vi "SO-PPSU TDK Lambda Voltage update.vi"(7 "queue In":refnum<queue>, 8 "error In":errorcluster, 9 "Ramp  time(sec)":dbl, 10 "connection ID":refnum<k5>, 11 "Voltage":string) -> (0 "error out":errorcluster, 1 "Boolean":bool, 2 "connection ID 3":refnum<k5>, 4 "PPSU OUT PUT":T1, 5 "queue In 2":refnum<queue>)   [LabVIEW 2022 SP3]
uses:
  <vilib>/ptbypt/NI_PtbyPt.lvlib
  <vilib>/Analysis/NI_AALBase.lvlib
  Controls/FGV Read write.ctl
  <vilib>/Analysis/1siggen.llb/Ramp Pattern by Samples.vi
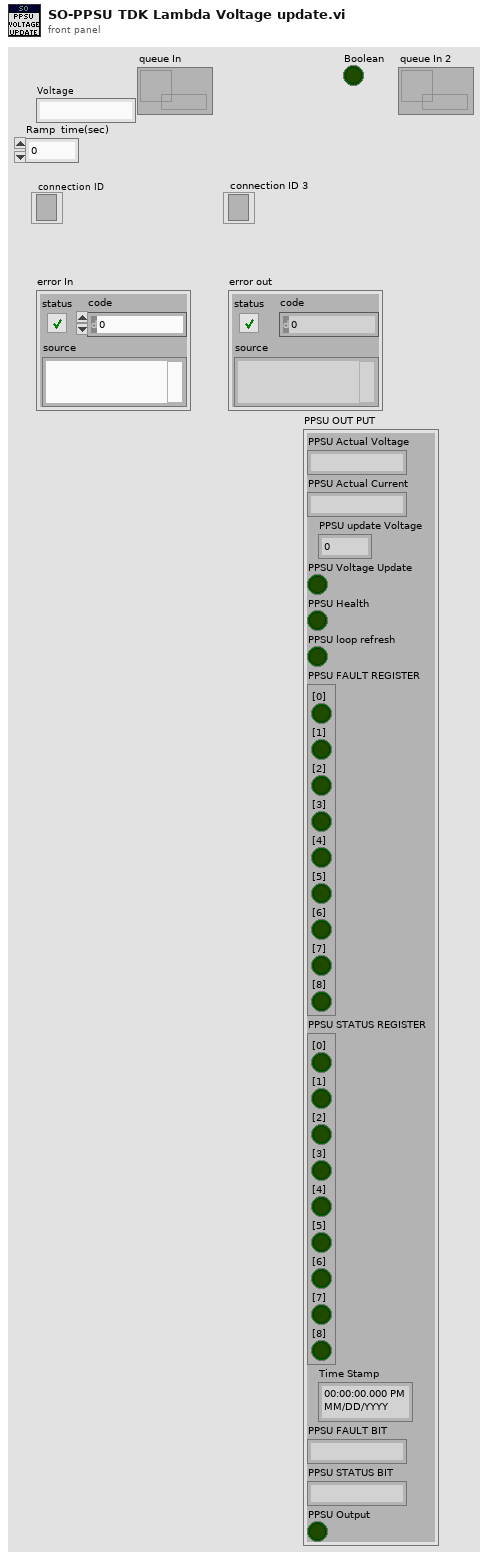
[diagram p1: front panel]
types:
  T1 = cluster{"PPSU Actual Voltage ":string, "PPSU Actual Current ":string, "PPSU update Voltage ":dbl, "PPSU Voltage Update":bool, "PPSU Health":bool, "PPSU loop refresh":bool, "PPSU FAULT REGISTER":cluster{"[0]":bool, "[1]":bool, "[2]":bool, "[3]":bool, "[4]":bool, "[5]":bool, "[6]":bool, "[7]":bool, "[8]":bool}, "PPSU STATUS REGISTER":cluster{"[0]":bool, "[1]":bool, "[2]":bool, "[3]":bool, "[4]":bool, "[5]":bool, "[6]":bool, "[7]":bool, "[8]":bool}, "Time Stamp":timestamp, "PPSU FAULT BIT":string, "PPSU STATUS BIT ":string, "PPSU Output":bool}
  T2 = typedef "FGV Read write.ctl" = enum16{"Write", "Read"}
  T3 = cluster{"[0]":bool, "[1]":bool, "[2]":bool, "[3]":bool, "[4]":bool, "[5]":bool, "[6]":bool, "[7]":bool, "[8]":bool}
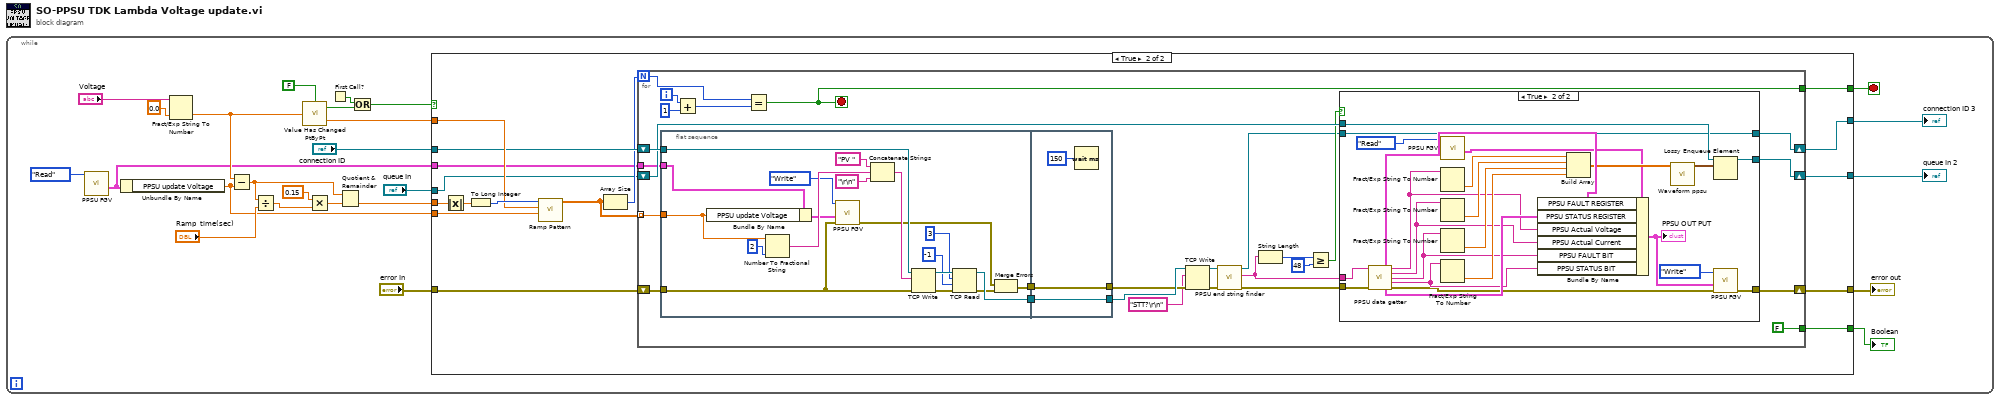
[diagram p0: block diagram]
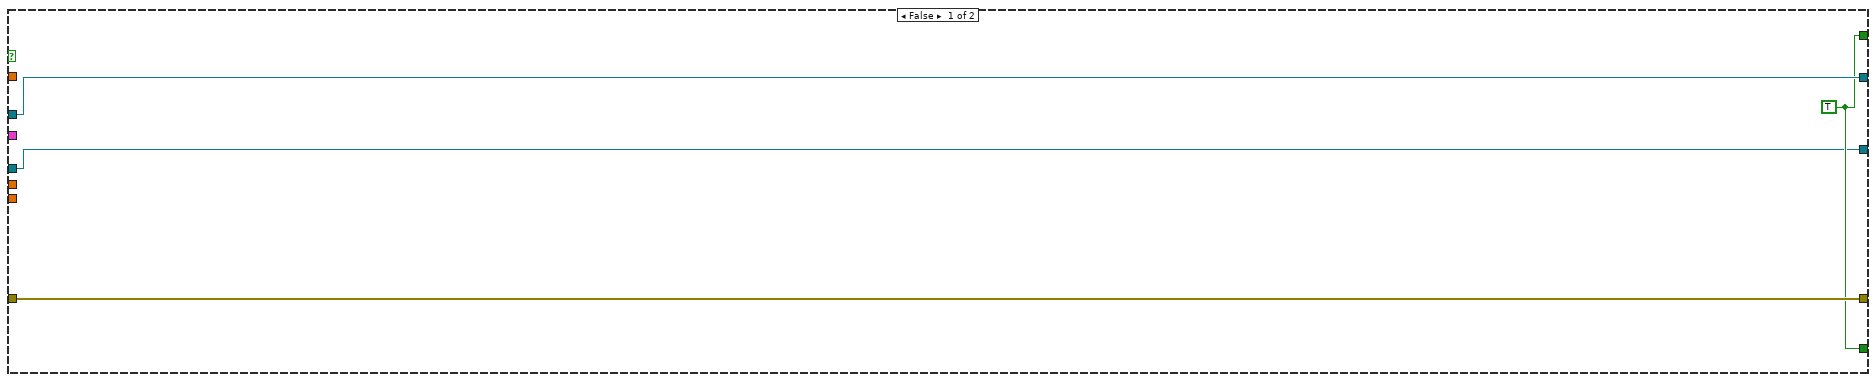
[diagram p2: hidden frame]
diagram:
  n1 = while {
    stop <- w8 stop-if-true
    n2 = call "PPSU FGV.vi"("Write/Read"=FGV_Read_write."Read") -> ("PPSU (R)"=w1:T1)  [unwired: 9 in, 1 out]
    n3 = Unbundle By Name(w1) -> ("PPSU update Voltage"=w2:dbl)
    n4 = Fract/Exp String To Number(string="Voltage", default (0 dbl)=0.0) -> (number=w12:dbl)  [unwired: 2 in, 1 out]
    n5 = Subtract(x=w12, y=w2) -> (x-y=w11:dbl)
    n6 = Divide(x=w11, y="Ramp  time(sec)") -> (x/y=w5:dbl)
    n7 = call <vilib>:"Value Has Changed PtByPt.vi"("input data point"=w12, "initialize"=FALSE) -> ("has changed"=w18:bool, "output data point"=w15:dbl)
    n8 = Multiply(x=0.15, y=w5) -> (x*y=w4:dbl)
    n9 = First Call?() -> (First Call?: T/F=w19:bool)
    n10 = Quotient & Remainder(x=w11, y=w4) -> (floor(x/y)=w16:dbl)  [unwired: 1 out]
    n11 = Or(x=w19, y=w18) -> (x .or. y?=w17:bool)
    n12 = case shown="True" w17 {
      tunnel: w16 -> [_ w45]
      tunnel: w15 -> [_ w42]
      tunnel: w2 -> [_ w41]
      tunnel: "connection ID" -> [w29 w39]
      tunnel: "error In" -> [w28 w38]
      tunnel: [w29 w37] -> w22
      tunnel: [w28 w36] -> w21
      tunnel: [w27 w34] -> w13
      tunnel: [w27 w33] -> w8
      tunnel: "queue In" -> [w26 w32]
      tunnel: [w26 w31] -> w6
      tunnel: w1 -> [_ w30]
      frame False {
        w27 = TRUE
      }
      frame True {
        n13 = Absolute Value(x=w45) -> (abs(x)=w44:dbl)
        n14 = To Long Integer(number=w44) -> (32bit integer=w43:i32)
        n15 = call-poly <vilib>:"Ramp Pattern.vi"("start"=w41, "end"=w42, "samples"=w43) -> ("Ramp Pattern"=w40:dbl[])  [unwired: 7 in, 1 out]
        n16 = Array Size(array=w40) -> (size(s)=w35:i32)
        n17 = for {
          N: w35 -> [w68]
          tunnel: w40 -> [w70] mode=indexing
          shift-right: [w47] -> w37
          shift-left: w39 -> [w72]
          shift-right: [w56] -> w36
          shift-left: w38 -> [w71]
          tunnel: [FALSE] -> w34
          tunnel: [w64] -> w33
          shift-right: [w57] -> w31
          shift-left: w32 -> [w58]
          tunnel: w30 -> [w46]
          i -> [w67]
          stop <- w64 stop-if-true
          n18 = flat-sequence {
            tunnel: w72 -> [w117]
            tunnel: w71 -> [w103]
            tunnel: w70 -> [w99]
            tunnel: [w108] -> w61
            tunnel: [w105] -> w60
            tunnel: w46 -> [w101]
            tunnel: [w119] -> w62
            tunnel: [w120] -> w63
            tunnel: w61 -> [w120]
            tunnel: w60 -> [w119]
            frame #0 {
              n19 = Bundle By Name(cluster=w101, "PPSU update Voltage"=w99) -> (w100:T1)
              n20 = Number To Fractional String(number=w99, precision (6)=i16 2) -> (F-format string=w113:string)  [unwired: 2 in]
              n21 = call "PPSU FGV.vi"("error in"=w103, "PPSU (W)"=w100, "Write/Read"=FGV_Read_write."Write") -> ("error out"=w102:errorcluster)  [unwired: 7 in, 1 out]
              n22 = Concatenate Strings("PV " ("string"), w113, "\r\n" ("string")) -> (w112:string)
              n23 = TCP Write(connection ID=w117, data in=w112, error in (no error)=w103) -> (connection ID out=w111:refnum<k5>, error out=w110:errorcluster)  [unwired: 1 in, 1 out]
              n24 = TCP Read(connection ID=w111, bytes to read=3, error in (no error)=w110, 9:-1 ("timeout ms (25000)")) -> (connection ID out=w108:refnum<k5>, error out=w106:errorcluster)  [unwired: 1 in, 1 out]
              n25 = Merge Errors(w102, w106) -> (w105:errorcluster)
            }
            frame #1 {
              n26 = Wait (ms)(milliseconds to wait=u32 150) -> ()  [unwired: 1 out]
            }
          }
          n27 = Add(x=w67, y=1) -> (x+y=w65:i32)
          n28 = Equal?(x=w68, y=w65) -> (x = y?=w64:bool)
          n29 = TCP Write(connection ID=w63, data in="STT?\r\n", error in (no error)=w62) -> (connection ID out=w54:refnum<k5>, error out=w53:errorcluster)  [unwired: 1 in, 1 out]
          n30 = call "PPSU end string finder.vi"("error in (no error)"=w53, "TCP Network Connection in"=w54) -> ("error out"=w59:errorcluster, "String"=w52:string, "TCP Network Connection out"=w48:refnum<k5>)  [unwired: 7 in]
          n31 = String Length(string=w52) -> (length=w50:i32)
          n32 = Greater Or Equal?(x=w50, y=48) -> (x >= y?=w51:bool)
          n33 = case shown="True" w51 {
            tunnel: w59 -> [w74 w95]
            tunnel: w58 -> [w75 w94]
            tunnel: [w75 w93] -> w57
            tunnel: [w74 w80] -> w56
            tunnel: w52 -> [_ w79]
            tunnel: w48 -> [w73 w78]
            tunnel: [w73 w78] -> w47
            frame False {
            }
            frame True {
              n34 = call "PPSU data getter.vi"("data in"=w79, "error in"=w95) -> ("FAULT"=w97:T3, "Voltage PPSU"=w87:string, "Current PPSU"=w86:string, "Fault"=w85:string, "status"=w84:string, "STATUS"=w98:T3, "error in  2"=w81:errorcluster)  [unwired: 7 in]
              n35 = call "PPSU FGV.vi"("Write/Read"=FGV_Read_write."Read") -> ("PPSU (R)"=w76:T1)  [unwired: 9 in, 1 out]
              n36 = Fract/Exp String To Number(string=w87) -> (number=w91:dbl)  [unwired: 3 in, 1 out]
              n37 = Fract/Exp String To Number(string=w86) -> (number=w90:dbl)  [unwired: 3 in, 1 out]
              n38 = Fract/Exp String To Number(string=w85) -> (number=w89:dbl)  [unwired: 3 in, 1 out]
              n39 = Fract/Exp String To Number(string=w84) -> (number=w88:dbl)  [unwired: 3 in, 1 out]
              n40 = Bundle By Name(cluster=w76, "PPSU FAULT REGISTER"=w97, "PPSU STATUS REGISTER"=w98, "PPSU Actual Voltage"=w87, "PPSU Actual Current"=w86, "PPSU FAULT BIT"=w85, "PPSU STATUS BIT"=w84) -> (w82:T1)
              "PPSU OUT PUT" <- w82
              n41 = Build Array(w91, w90, w89, w88) -> (w83:dbl[])
              n42 = call "Waveform ppsu.vi"("Array in"=w83) -> ("Array out"=w92:waveform(dbl)[])  [unwired: 10 in]
              n43 = Lossy Enqueue Element(queue=w94, element=w92) -> (queue out=w93:refnum<queue>)  [unwired: 1 in, 3 out]
              n44 = call "PPSU FGV.vi"("error in"=w81, "PPSU (W)"=w82, "Write/Read"=FGV_Read_write."Write") -> ("error out"=w80:errorcluster)  [unwired: 7 in, 1 out]
            }
          }
        }
      }
    }
    "connection ID 3" <- w22
    "error out" <- w21
    "Boolean" <- w13
    "queue In 2" <- w6
  }
